vi "Initialize.vi"(8 "error in (no error)":errorcluster caption="错误输入（无错误）", 10 "Reset? (T: Reset)":bool=TRUE, 11 "TH6402 输入":refnum<class "TH6402.lvclass">) -> (0 "error out":errorcluster caption="错误输出", 3 "TH6402 输出":refnum<class "TH6402.lvclass">)   [LabVIEW 2020, in "DP.lvlib" / "TH6402.lvclass"]
uses:
  TH6402.lvclass
  D:/LVProject/Class/LVDevClass/DP/root/DP.lvclass
  TH6402.lvclass/TH6402.ctl
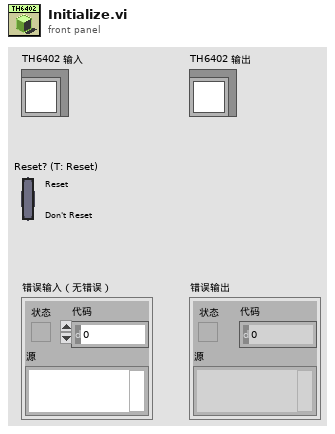
[diagram p1: front panel]
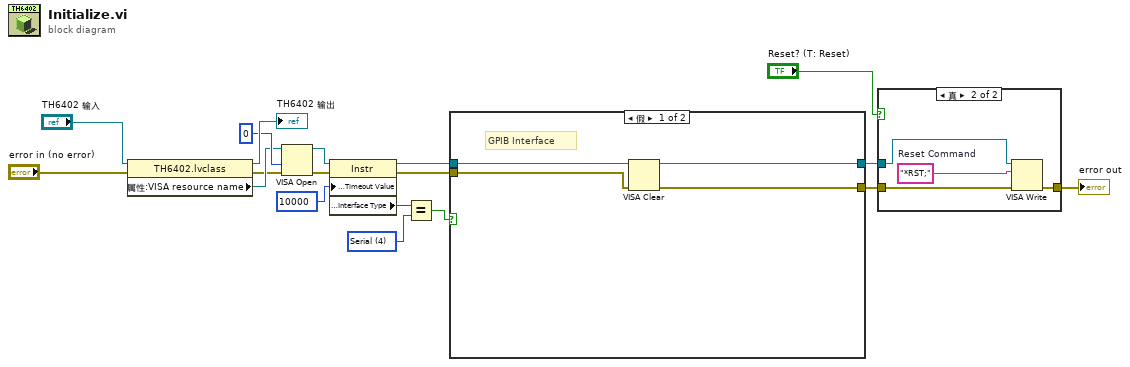
[diagram p0: block diagram]
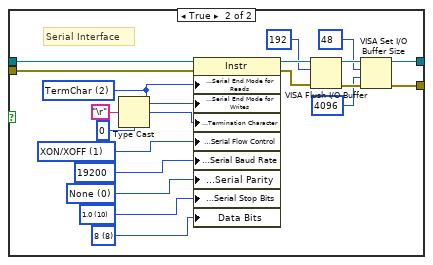
[diagram p3: hidden frame]
diagram:
  w12 = u16 4 items=["GPIB"=1, "VXI"=2, "GPIB-VXI"=3, "Serial"=4, "PXI"=5, "TCPIP"=6, "USB"=7] ("Interface Information:Interface Type")
  n1 = property class="TH6402.lvclass"(reference="TH6402 输入", error in="error in (no error)") -> (reference out=→"TH6402 输出":refnum<class "TH6402.lvclass">, error out=w5:errorcluster, "属性:VISA resource name"=w6:refnum<visa-resource-name>)
  n2 = VISA Open(access mode=u32 0, error in (no error)=w5, VISA resource name=w6) -> (VISA resource name=w14:refnum<visa-resource-name>, error out=w15:errorcluster)  [unwired: 2 in]
  n3 = property class="Instr"(reference=w14, error in=w15, "General Settings:Timeout Value"=u32 10000) -> (reference out=w9:refnum<visa-resource-name>, error out=w10:errorcluster, "Interface Information:Interface Type"=w7:u16)
  n4 = Equal?(x=w7, y=w12) -> (x = y?=w11:bool)
  n5 = case shown="假" w11 {
    tunnel: [w20 w39] -> w1
    tunnel: [w19 w36] -> w4
    tunnel: w9 -> [w22 w41]
    tunnel: w10 -> [w21 w42]
    frame False {
      # "GPIB Interface"
      n6 = VISA Clear(VISA resource name=w22, error in (no error)=w21) -> (VISA resource name out=w20:refnum<visa-resource-name>, error out=w19:errorcluster)
    }
    frame True {
      w23 = u16 8 items=["7"=7, "8"=8] ("Data Bits")
      w24 = u16 10 items=["1.0"=10, "1.5"=15, "2.0"=20] ("Serial Settings:Serial Stop Bits")
      w27 = u16 0 items=["None", "Odd", "Even", "Mark", "Space"] ("Serial Settings:Serial Parity")
      w29 = u16 2 items=["None", "LastBit", "TermChar"] ("Serial Settings:Serial End Mode for Reads")
      w25 = u16 1 items=["None"=0, "XON/XOFF"=1, "RTS/CTS"=2, "DTR/DSR"=4] ("Serial Settings:Serial Flow Control")
      # "Serial Interface"
      n7 = Type Cast(type=u8 0, x="\r") -> (*(type *) &x=w28:u8)
      n8 = property class="Instr"(reference=w41, error in=w42, "Serial Settings:Serial End Mode for Reads"=w29, "Serial Settings:Serial End Mode for Writes"=w29, "Message Based Settings:Termination Character"=w28, "Serial Settings:Serial Flow Control"=w25, "Serial Settings:Serial Baud Rate"=u32 19200, "Serial Settings:Serial Parity"=w27, "Serial Settings:Serial Stop Bits"=w24, "Data Bits"=w23) -> (reference out=w35:refnum<visa-resource-name>, error out=w38:errorcluster)
      n9 = VISA Flush I/O Buffer(VISA resource name=w35, mask (16)=u16 192, error in (no error)=w38) -> (VISA resource name out=w40:refnum<visa-resource-name>, error out=w37:errorcluster)
      n10 = VISA Set I/O Buffer Size(VISA resource name=w40, mask (16)=u16 48, size (4096)=u32 4096 ("size (0)"), error in (no error)=w37) -> (VISA resource name out=w39:refnum<visa-resource-name>, error out=w36:errorcluster)
    }
  }
  n11 = case shown="真" "Reset? (T: Reset)" {
    tunnel: w4 -> [w43 w47]
    tunnel: [w43 w46] -> w3
    tunnel: w1 -> [_ w44]
    frame False {
    }
    frame True {
      w45 = "*RST;"  # Reset Command
      n12 = VISA Write(VISA resource name=w44, write buffer=w45, error in (no error)=w47) -> (error out=w46:errorcluster)  [unwired: 2 out]
    }
  }
  "error out" <- w3
